vi "_s_Look for serial devices.vi"(7 "Comunicaciones":T1={"Flujo_1"="COM4", "Brk1"=TRUE, "Flujo_2"="COM6", "Brk2"=TRUE, "Flujo_3"="COM8", "Brk3"=TRUE, "Flujo_4"="COM10", "Brk4"=TRUE, "Eurothe"="COM23", "Eurot"=FALSE, "Balanza"="COM24", "Bal"=FALSE, "eValPos"="COM25", "eVal"=FALSE, "flowbus"="COM26", "fb"=FALSE}, 8 "error in (no error)":errorcluster) -> (0 "error out":errorcluster, 3 "Dispositivos":T2=[["3", "NO", "M0000013", "Air", "1", "ln/mn", "0.1", "0.11"], ["4", "NO", "M0000014", "Air", "1", "ln/mn", "0.2", "0.22"], ["5", "NO", "M0000015", "Air", "1", "ln/mn", "0.3", "0.33"], ["6", "NO", "M0000016", "Air", "1", "ln/mn", "0.4", "0.44"], ["7", "NO", "M0000017", "Air", "1", "ln/mn", "0.5", "0.55"], ["8", "NO", "M0000018", "Air", "1", "ln/mn", "0.6", "0.66"], ["9", "NO", "M0000019", "Air", "1", "ln/mn", "0.7", "0.77"], ["10", "NO", "M0000020", "Air", "1", "ln/mn", "0.8", "0.88"], ["11", "NO", "M0000021", "Air", "1", "ln/mn", "0.9", "0.99"]] caption="Controladores de flujo SERIE")   [LabVIEW 2013]
uses:
  _s_TablaBronkhorst.ctl
  Controles/P2018 Com Control.ctl
  _s_Bronkhorst Control.ctl
panel:
  out "Address":i32
  in  "stop":bool
  out "Status":string
  # "Buscando controladores"
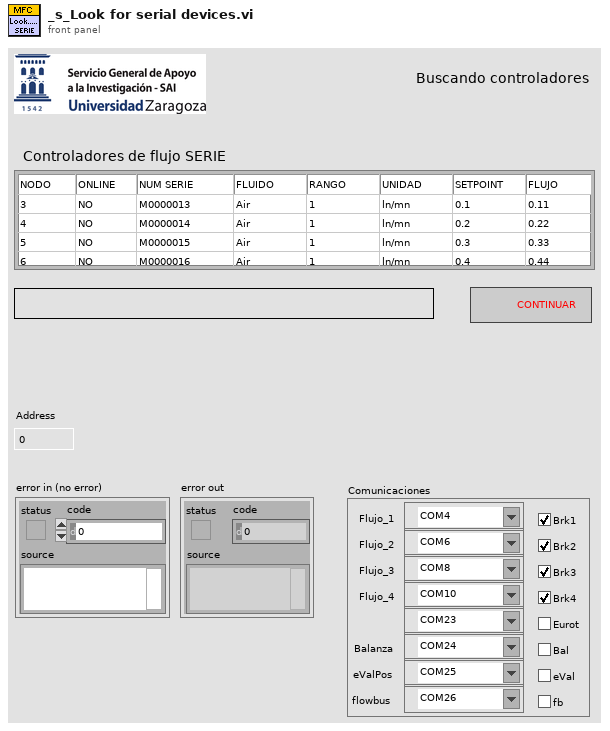
[diagram p1: front panel]
types:
  T1 = typedef "P2018 Com Control.ctl" = cluster{"Flujo_1":refnum<visa-resource-name>, "Brk1":bool, "Flujo_2":refnum<visa-resource-name>, "Brk2":bool, "Flujo_3":refnum<visa-resource-name>, "Brk3":bool, "Flujo_4":refnum<visa-resource-name>, "Brk4":bool, "Eurothe":refnum<visa-resource-name>, "Eurot":bool, "Balanza":refnum<visa-resource-name>, "Bal":bool, "eValPos":refnum<visa-resource-name>, "eVal":bool, "flowbus":refnum<visa-resource-name>, "fb":bool}
  T2 = typedef "_s_TablaBronkhorst.ctl" = string[][]
  T3 = typedef "_s_Bronkhorst Control.ctl" = enum16{"Inicializar", "Request IdnString", "Request Serial Number", "Request Fluid Number", "Request Fluid Name", "Request Sensor Type", "Request Cap 0", "Request Cap100", "Request Units", "Request CapUnitStr", "Request Setpoint %", "Request Setpoint", "Request Measure %", "Request Measure ", "Send Control Mode", "Send Fluid Number", "Send Setpoint %", "Send Setpoint", "Shutdown"}
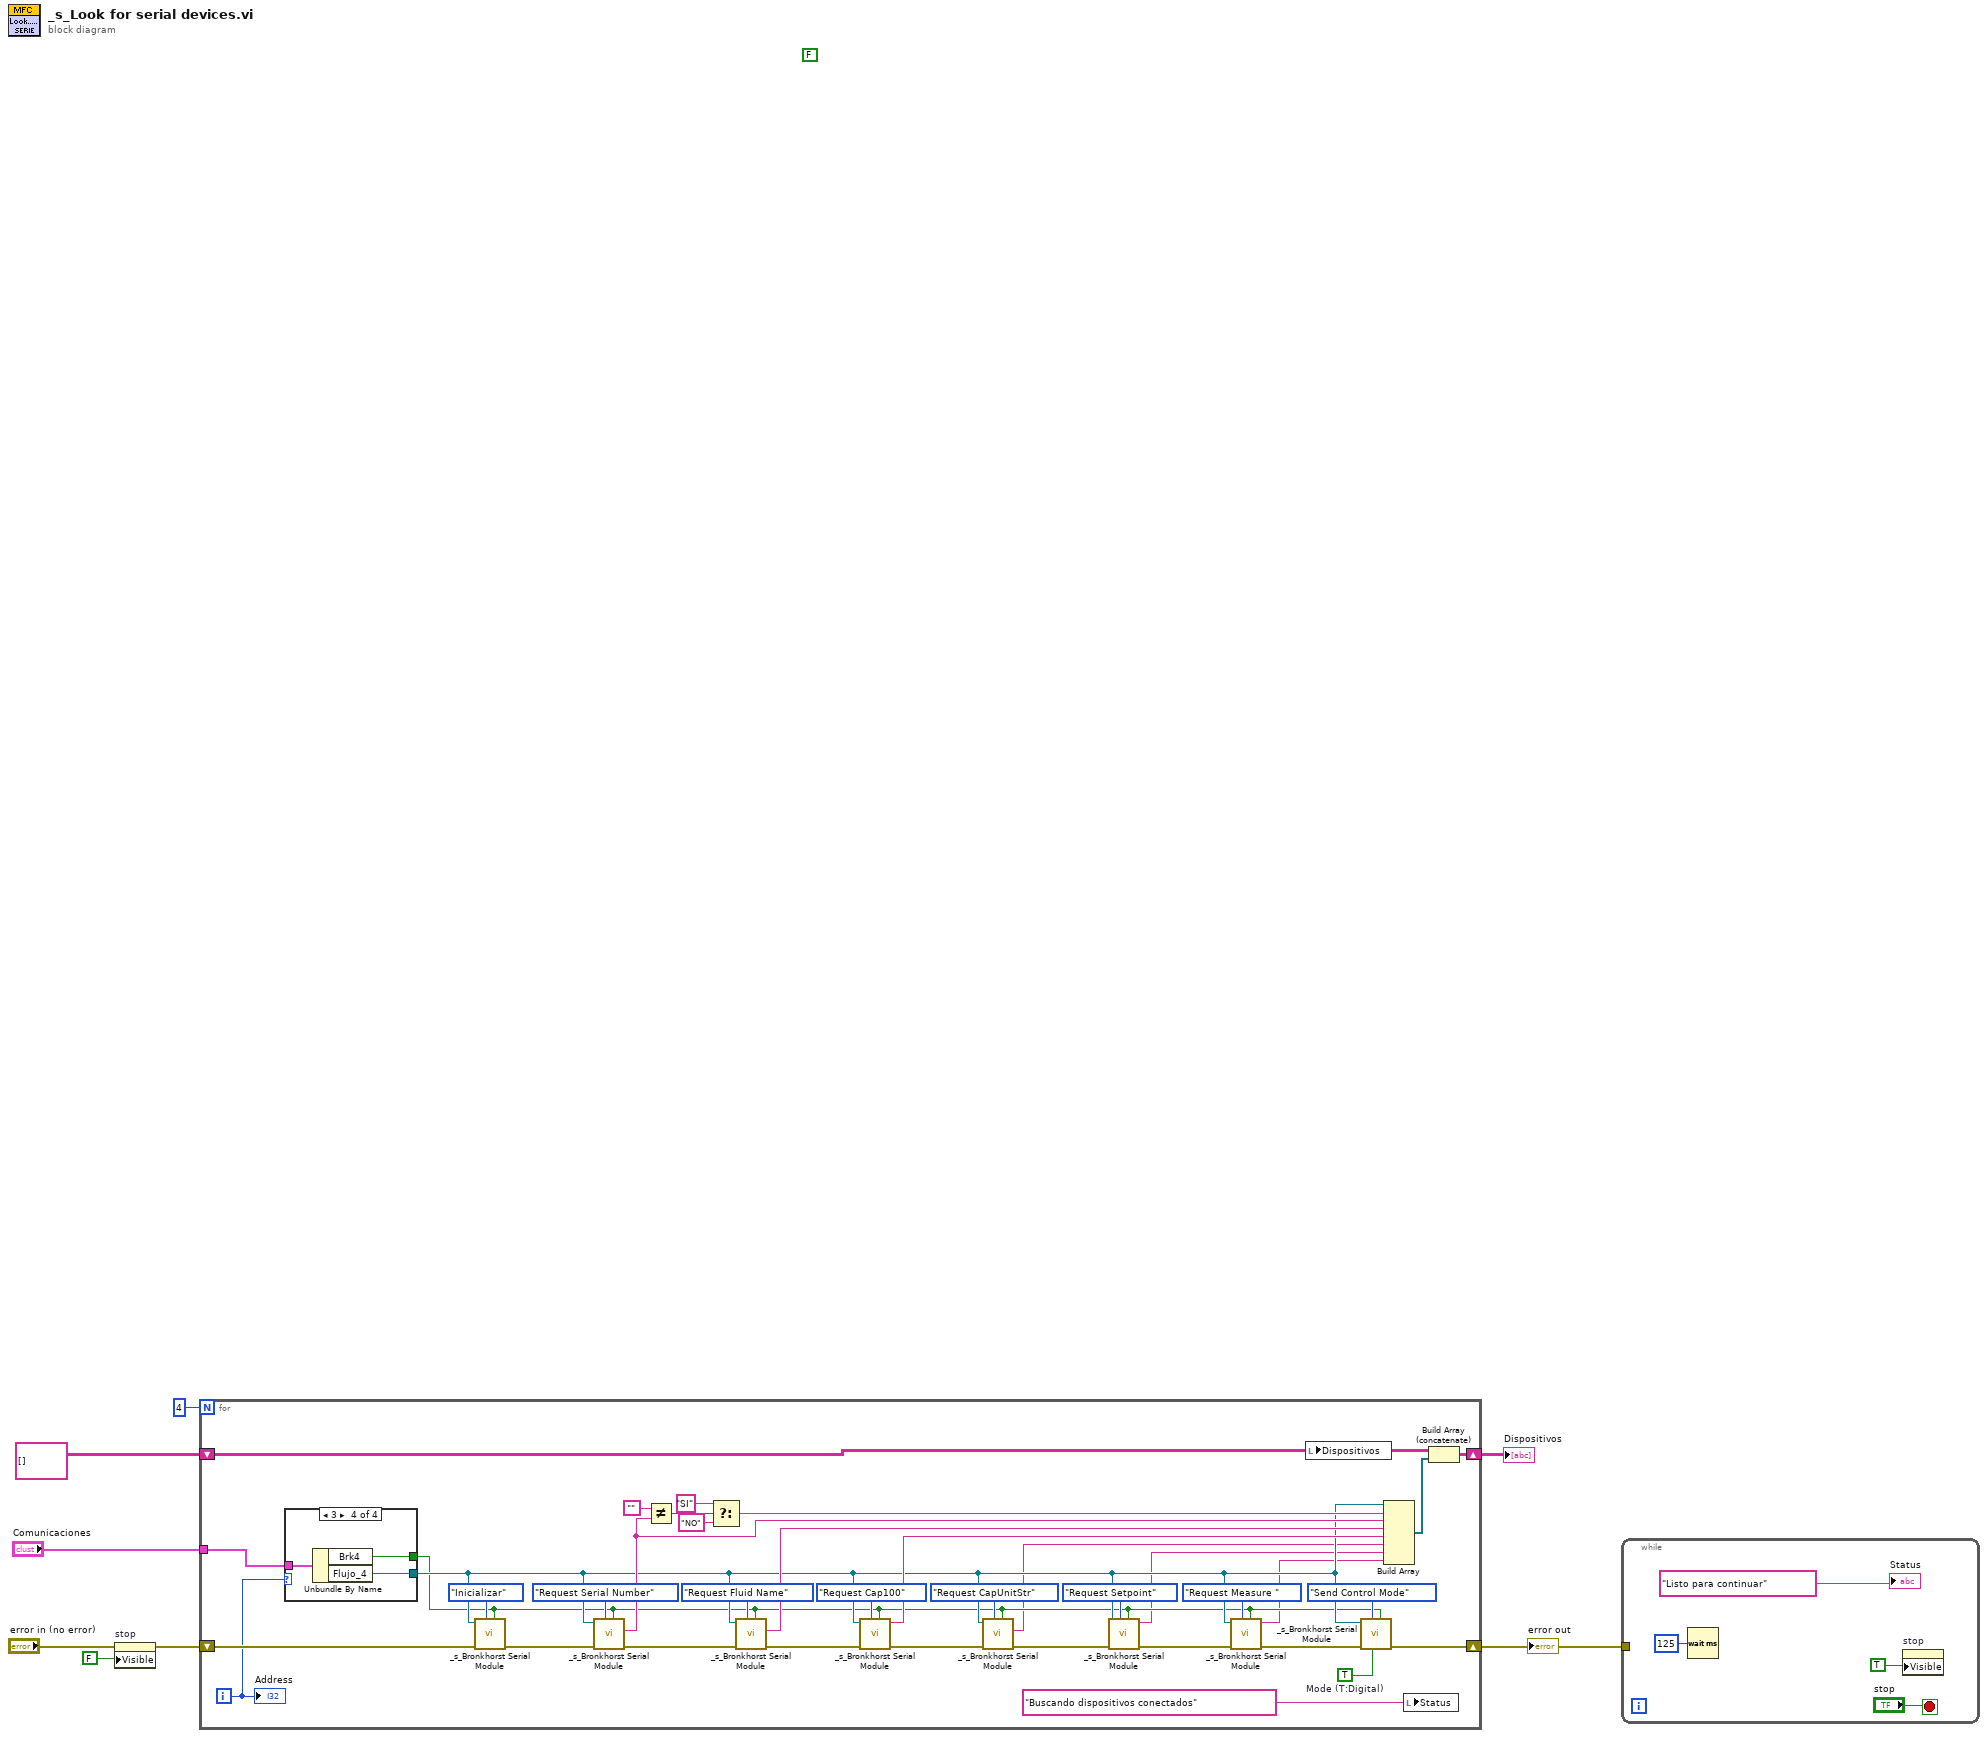
[diagram p0: block diagram]
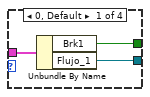
[diagram p2: hidden frame]
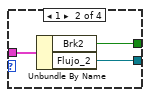
[diagram p3: hidden frame]
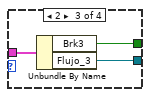
[diagram p4: hidden frame]
diagram:
  (unwired) FALSE
  n1 = property on="stop" class="Bool"(error in="error in (no error)", "Visible"=FALSE) -> (error out=w6:errorcluster)  [unwired: 1 in, 1 out]
  n2 = for {
    N: 4 -> [_]
    shift-right: [w18] -> w5
    shift-left: w6 -> [w26]
    tunnel: "Comunicaciones" -> [w25]
    shift-right: [w21] -> w1
    shift-left: string[][] [] -> [w20]
    i -> [w24]
    w17 = TRUE  # Mode (T:Digital)
    n3 = case shown="3" w24 {
      tunnel: w25 -> [w48 w51 w54 w57]
      tunnel: [w47 w50 w53 w56] -> w12
      tunnel: [w46 w49 w52 w55] -> w16
      frame 0, Default {
        n4 = Unbundle By Name(w48) -> ("Brk1"=w47:bool, "Flujo_1"=w46:refnum<visa-resource-name>)
      }
      frame 1 {
        n5 = Unbundle By Name(w51) -> ("Brk2"=w50:bool, "Flujo_2"=w49:refnum<visa-resource-name>)
      }
      frame 2 {
        n6 = Unbundle By Name(w54) -> ("Brk3"=w53:bool, "Flujo_3"=w52:refnum<visa-resource-name>)
      }
      frame 3 {
        n7 = Unbundle By Name(w57) -> ("Brk4"=w56:bool, "Flujo_4"=w55:refnum<visa-resource-name>)
      }
    }
    n8 = call "_s_Bronkhorst Serial Module.vi"("Module (T:Enable)"=w12, "Command"=_s_Bronkhorst_Control."Inicializar", "error in (no error)"=w26, "VISA resource name"=w16) -> ("error out"=w43:errorcluster)  [unwired: 4 in, 3 out]
    n9 = call "_s_Bronkhorst Serial Module.vi"("Module (T:Enable)"=w12, "Command"=_s_Bronkhorst_Control."Request Serial Number", "error in (no error)"=w43, "VISA resource name"=w16) -> ("error out"=w32:errorcluster, "Result"=w37:string)  [unwired: 4 in, 2 out]
    n10 = Not Equal?(x="", y=w37) -> (x != y?=w42:bool)
    n11 = Select(t="SI", s=w42, f="NO") -> (s? t:f=w39:string)
    n12 = call "_s_Bronkhorst Serial Module.vi"("Module (T:Enable)"=w12, "Command"=_s_Bronkhorst_Control."Request Fluid Name", "error in (no error)"=w32, "VISA resource name"=w16) -> ("error out"=w30:errorcluster, "Result"=w31:string)  [unwired: 4 in, 2 out]
    n13 = call "_s_Bronkhorst Serial Module.vi"("Module (T:Enable)"=w12, "Command"=_s_Bronkhorst_Control."Request Cap100", "error in (no error)"=w30, "VISA resource name"=w16) -> ("error out"=w29:errorcluster, "Value"=w27:string)  [unwired: 4 in, 2 out]
    n14 = call "_s_Bronkhorst Serial Module.vi"("Module (T:Enable)"=w12, "Command"=_s_Bronkhorst_Control."Request CapUnitStr", "error in (no error)"=w29, "VISA resource name"=w16) -> ("error out"=w28:errorcluster, "Result"=w9:string)  [unwired: 4 in, 2 out]
    n15 = call "_s_Bronkhorst Serial Module.vi"("Module (T:Enable)"=w12, "Command"=_s_Bronkhorst_Control."Request Setpoint", "error in (no error)"=w28, "VISA resource name"=w16) -> ("error out"=w14:errorcluster, "Value"=w11:string)  [unwired: 4 in, 2 out]
    n16 = call "_s_Bronkhorst Serial Module.vi"("Module (T:Enable)"=w12, "Command"=_s_Bronkhorst_Control."Request Measure ", "error in (no error)"=w14, "VISA resource name"=w16) -> ("error out"=w13:errorcluster, "Value"=w10:string)  [unwired: 4 in, 2 out]
    n17 = local write "Dispositivos"(w20) -> ()
    n18 = call "_s_Bronkhorst Serial Module.vi"("Module (T:Enable)"=w12, "Mode (T:Digital)"=w17, "Command"=_s_Bronkhorst_Control."Send Control Mode", "error in (no error)"=w13, "VISA resource name"=w16) -> ("error out"=w18:errorcluster)  [unwired: 3 in, 3 out]
    n19 = Build Array(w16, w39, w37, w31, w27, w9, w11, w10) -> (w22:refnum<visa-resource-name>[])
    n20 = local write "Status"("Buscando dispositivos conectados" ("Status")) -> ()
    n21 = Build Array (concatenate)(w20, w22) -> (w21:string[][])
    "Address" <- w24
  }
  "error out" <- w5
  "Dispositivos" <- w1
  n22 = while {
    tunnel: w5 -> [_]
    stop <- "stop" stop-if-true
    n23 = Wait (ms)(milliseconds to wait=u32 125) -> ()  [unwired: 1 out]
    n24 = property on="stop" class="Bool"("Visible"=TRUE) -> ()  [unwired: 2 in, 2 out]
    "Status" <- "Listo para continuar" ("Status")
  }
